vi "getAOwfm.vi"(8 "error in (no error)":errorcluster, 11 "Instrument.LockinAPI in":refnum<class "Instrument.LockinAPI.lvclass">) -> (0 "error out":errorcluster, 2 "AO Waveforrm":waveform(dbl)[](array[waveform]), 3 "Instrument.LockinAPI out":refnum<class "Instrument.LockinAPI.lvclass">)   [LabVIEW 2019, in "Instrument.LockinAPI.lvclass"]
doc: "API to get the AO waveforms.\n\nIf address=\"\", this API reads from localhost\nIf address is remote lockin, you need to add this computer to allowed whitelist on the lockin computer you are trying to access."
uses:
  Instrument.LockinAPI.lvclass
  C:/Users/patrick/Documents/GitHub/Instrument-Framework/lvsrc/Instrument/Instrument.lvclass
  Typedefs/API/LockinAPI.Commands--Enum.ctl
  a13456fa-5815-4e62-a9ee-67b49defb4d3.vi
  a13456fa-5815-4e62-a9ee-67b49defb4d3.vi/134e3a92-4866-447c-8482-174aac171cb3.vi
  a13456fa-5815-4e62-a9ee-67b49defb4d3.vi/134e3a92-4866-447c-8482-174aac171cb3.vi/193dc0d4-fccd-436a-b502-7a84f1b6c134.vi
  a13456fa-5815-4e62-a9ee-67b49defb4d3.vi/134e3a92-4866-447c-8482-174aac171cb3.vi/b0f1922e-1d8a-438a-b361-78db954e47f2.vi
  a13456fa-5815-4e62-a9ee-67b49defb4d3.vi/134e3a92-4866-447c-8482-174aac171cb3.vi/05f5b1b1-709d-4ca1-b4d7-5d0c421112cb.vi
  <vilib>/JDP Science/JSONtext/Make JSON Array.vi
  a13456fa-5815-4e62-a9ee-67b49defb4d3.vi/134e3a92-4866-447c-8482-174aac171cb3.vi/b0f1922e-1d8a-438a-b361-78db954e47f2.vi/670806cf-2cac-44de-9167-4d6c8a2eff4c.vi
  a13456fa-5815-4e62-a9ee-67b49defb4d3.vi/134e3a92-4866-447c-8482-174aac171cb3.vi/05f5b1b1-709d-4ca1-b4d7-5d0c421112cb.vi/86e764e1-b441-461a-bf38-126408ba43ef.vi
  a13456fa-5815-4e62-a9ee-67b49defb4d3.vi/134e3a92-4866-447c-8482-174aac171cb3.vi/05f5b1b1-709d-4ca1-b4d7-5d0c421112cb.vi/ada29d68-b3de-4174-acba-089ece6cb446.vi
  Instrument/API/Enum to String.vi
  Instrument/Private/Get RC Connection Status.vi
  <vilib>/JDP Science/JSONtext/Variant to JSON Text.vi
  <vilib>/JDP Science/JSONtext/support/Format JSON Array Text.vi
  Instrument/API/Send and Receive.vi
  <vilib>/JDP Science/JSONtext/JSON text to Variant.vi
  <vilib>/Utility/Data Type/Get Type Information.vi
  <vilib>/JDP Science/JSONtext/LVClass Serializer/JSONtext LVClass Serializer.lvclass
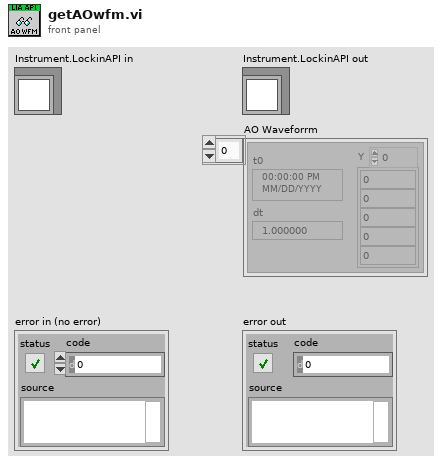
[diagram p1: front panel]
types:
  T1 = typedef "Instrument.LockinAPI.lvclass/LockinAPI.Commands--Enum.ctl" = enum16{"setAI", "setAO", "setAO_Amplitude", "setAO_DC", "setAO_Frequency", "setAO_Phase", "setAO_Function", "setAO_I+", "setREF", "setREF_Frequency", "setREF_Phase", "setREF_TC", "setREF_Roll-Off", "setDAQ", "setSampling", "setOffset", "setState", "getState", "getAO", "getAI", "getResults", "getSampling", "getAOconfig", "getREFconfig", "setInputGain", "setOutputGain", "getInputGain", "getOutputGain", "setSamplingMode", "getSamplingMode", "setSweep", "setSweepTime", "setSweepTable", "getStatus", "getSweepResults", "getSweepWaveforms", "startSweep", "stopSweep", "setAUX", "getAUX"}
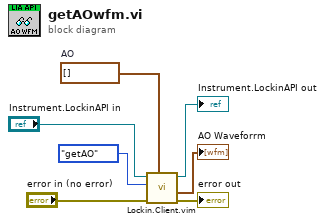
[diagram p0: block diagram]
diagram:
  w1 = waveform(dbl)[] []  # AO
  n1 = call "Lockin.Client.vim"("Data Out type"=w1, "error in (no error)"="error in (no error)", "Command"=LockinAPI.Commands--Enum."getAO", "Instrument.LockinAPI in"="Instrument.LockinAPI in") -> ("error out"=→"error out":errorcluster, "Data out"=→"AO Waveforrm":waveform(dbl)[], "Instrument.LockinAPI out"=→"Instrument.LockinAPI out":refnum<class "Instrument.LockinAPI.lvclass">)  [unwired: 5 in]
